vi "CUST Start Data Stream.vi"(11 "pseudoPdcId":i32) -> (3 "function return":i32)   [LabVIEW 2013, in "C37118-DLL.lvlib"]
doc: "STRONGRIDIEEEC37118DLL_API int __cdecl startDataStream( int32_t pseudoPdcId);"
uses:
  C37118-DLL.lvlib
  StrongridDLL/StrongridDLL.dll
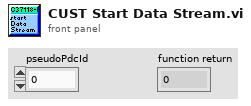
[diagram p1: front panel]
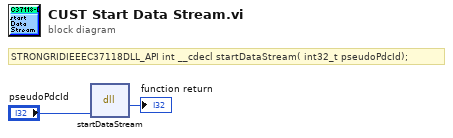
[diagram p0: block diagram]
diagram:
  # "STRONGRIDIEEEC37118DLL_API int __cdecl startDataStream( int32_t pseudoPdcId);"
  n1 = dll-call lib="C:/dev/OSS/S3DK/builds/StrongridDLL/StrongridDLL.*" fn="startDataStream"("pseudoPdcId"="pseudoPdcId") -> (→"function return":i32)  [unwired: 4 in, 2 out]
